vi "GetResult.vi"(0 "HttpBuff":string, 3 "error in (no error)":errorcluster caption="错误输入（无错误）", 4 "™z²é î‘B?":bool) -> (8 "î‘B":i32, 9 "”µ“þ":string, 10 "error out":errorcluster caption="错误输出")   [LabVIEW 2012, in "Http.lvclass"]
uses:
  Http.lvclass
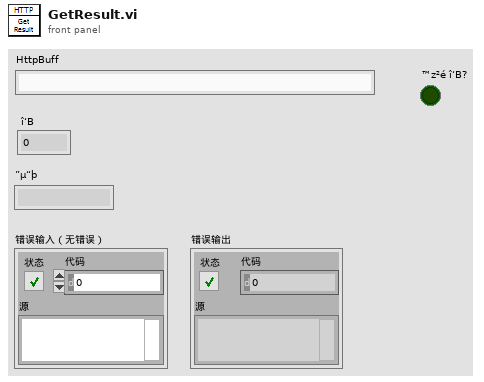
[diagram p1: front panel]
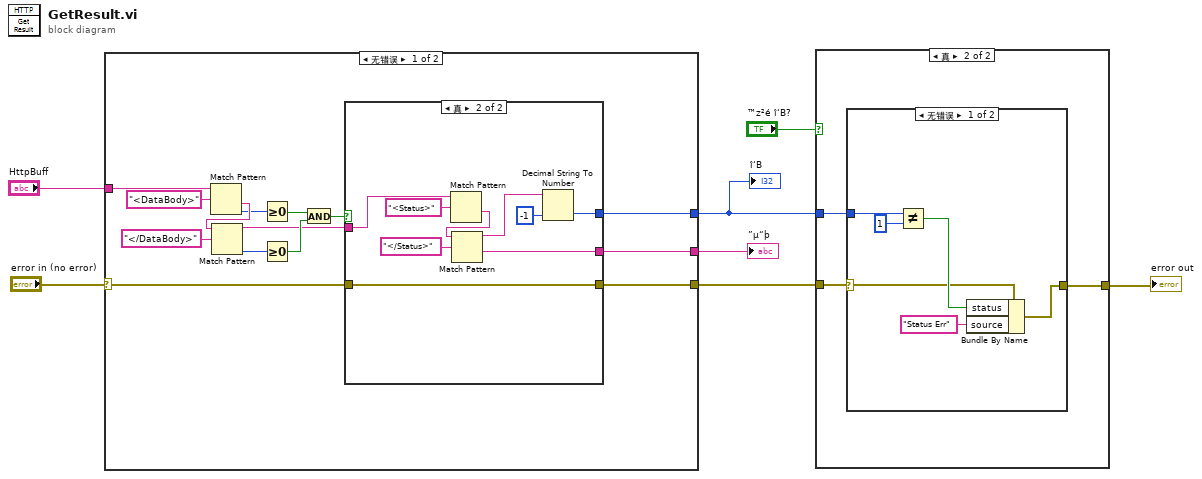
[diagram p0: block diagram]
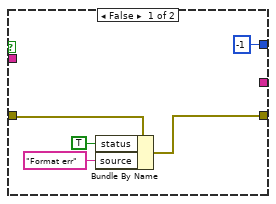
[diagram p4: hidden frame]
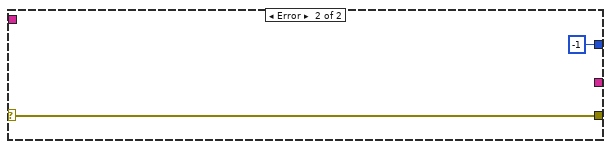
[diagram p5: hidden frame]
diagram:
  n1 = case shown="无错误" "error in (no error)" {
    selector: "error in (no error)" -> [w12 w36]
    tunnel: "HttpBuff" -> [w21 _]
    tunnel: [w10 -1] -> w2
    tunnel: [w9 w36] -> w3
    tunnel: [w8 _] -> w5
    frame No Error {
      n2 = Match Pattern(string=w21, regular expression="<DataBody>" ("正则表达式")) -> (after substring=w19:string, offset past match=w17:i32)  [unwired: 1 in, 2 out]
      n3 = Match Pattern(string=w19, regular expression="</DataBody>" ("正则表达式")) -> (before substring=w11:string, offset past match=w16:i32)  [unwired: 1 in, 2 out]
      n4 = Greater Or Equal To 0?(x=w17) -> (x >= 0?=w15:bool)
      n5 = Greater Or Equal To 0?(x=w16) -> (x >= 0?=w14:bool)
      n6 = And(x=w15, y=w14) -> (x .and. y?=w13:bool)
      n7 = case shown="真" w13 {
        tunnel: w12 -> [w26 w29]
        tunnel: w11 -> [_ w32]
        tunnel: [-1 w30] -> w10
        tunnel: [w22 w29] -> w9
        tunnel: [_ w27] -> w8
        frame False {
          n8 = Bundle By Name(cluster=w26, "status"=TRUE, "source"="Format err") -> (w22:errorcluster)
        }
        frame True {
          n9 = Match Pattern(string=w32, regular expression="<Status>" ("正则表达式")) -> (after substring=w34:string)  [unwired: 1 in, 3 out]
          n10 = Match Pattern(string=w34, regular expression="</Status>" ("正则表达式")) -> (before substring=w31:string, after substring=w27:string)  [unwired: 1 in, 2 out]
          n11 = Decimal String To Number(string=w31, default (0L)=-1 ("默认(0 I32)")) -> (number=w30:i32)  [unwired: 1 in, 1 out]
        }
      }
    }
    frame Error {
    }
  }
  "î‘B" <- w2
  "”µ“þ" <- w5
  n12 = case shown="真" "™z²é î‘B?" {
    tunnel: w3 -> [w38 w40]
    tunnel: w2 -> [_ w41]
    tunnel: [w38 w39] -> w1
    frame False {
    }
    frame True {
      n13 = case shown="无错误" w40 {
        selector: w40 -> [w43 w48]
        tunnel: w41 -> [w47 _]
        tunnel: [w42 w48] -> w39
        frame No Error {
          n14 = Not Equal?(x=w47, y=1) -> (x != y?=w44:bool)
          n15 = Bundle By Name(cluster=w43, "status"=w44, "source"="Status Err") -> (w42:errorcluster)
        }
        frame Error {
        }
      }
    }
  }
  "error out" <- w1
